vi "Go2XYZ (SubVI).vi"(0 ".NET Refnum in":refnum<k24>, 5 "Go to Coordinates":T2={"Go to X"=25.0, "Go to Y"=12.5, "Go to Z"=5.0}, 7 "Axis Speeds":T4={"X Speed"=25.0, "Y Speed"=12.5, "Z Speed"=5.0}, 11 "error in (no error)":errorcluster) -> (4 ".NET Refnum out":refnum<k24>, 6 "Final Position":T1, 14 "Initial Position":T3, 15 "error out":errorcluster)   [LabVIEW 2016]
uses:
  C:/Users/Aerotech/Documents/BNLStaveAssembly/Bin/Aerotech.A3200.dll
  Bin/Aerotech.A3200.dll
  Motion/EnableMultiple.vi
  Motion/MoveIncMultiple.vi
  Motion/WaitMultiple.vi
  Motion/DisableMultiple.vi
panel:
  out "Step Distance":dbl[](array[numeric])
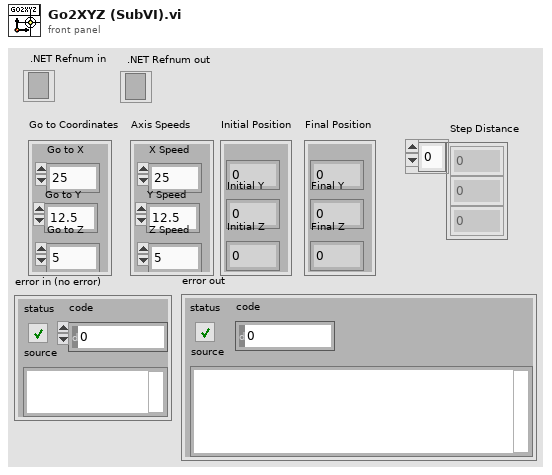
[diagram p1: front panel]
types:
  T1 = cluster{"Final X":dbl, "Final Y":dbl, "Final Z":dbl}
  T2 = cluster{"Go to X":dbl, "Go to Y":dbl, "Go to Z":dbl}
  T3 = cluster{"Initial X":dbl, "Initial Y":dbl, "Initial Z":dbl}
  T4 = cluster{"X Speed":dbl, "Y Speed":dbl, "Z Speed":dbl}
  T5 = cluster{"X Position Feedback":dbl, "Y Position Feedback":dbl, "Z Position Feedback":dbl}
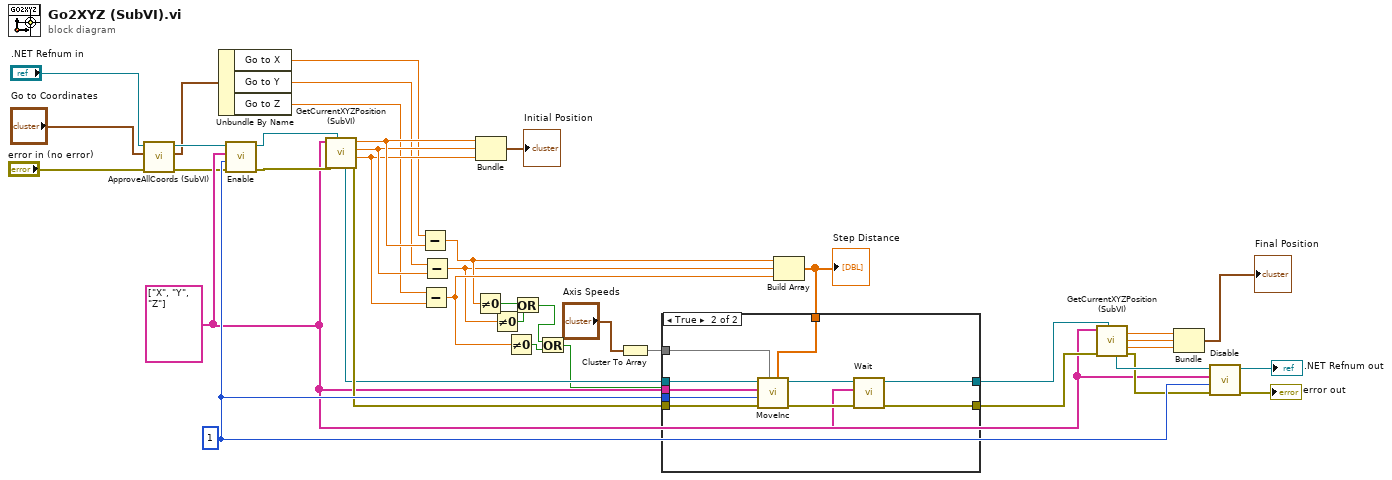
[diagram p0: block diagram]
diagram:
  w24 = string[] ["X", "Y", "Z"]
  w38 = 1 ("taskNumber")
  n1 = call "ApproveAllCoords (SubVI).vi"("error in (no error)"="error in (no error)", "Go to Coordinates"="Go to Coordinates", "Controller .NET Refnum in"=".NET Refnum in") -> ("error out"=w17:errorcluster, "Approved Coordinates"=w12:T2, "Controller .NET Refnum out"=w13:refnum<k24>)  [unwired: 6 in]
  n2 = Unbundle By Name(w12) -> ("Go to X"=w14:dbl, "Go to Y"=w15:dbl, "Go to Z"=w16:dbl)
  n3 = call-poly "Enable.vi"("error in (no error)"=w17, "taskId"=w38, "axis names"=w24, "controller in"=w13) -> ("error out"=w35:errorcluster, "controller out"=w34:refnum<k24>)  [unwired: 6 in]
  n4 = call "GetCurrentXYZPosition (SubVI).vi"(".NET Refnum in - Device"=w34, "error in (no error)"=w35, "Axes Names"=w24) -> ("error out"=w37:errorcluster, "Z Position Feedback"=w29:dbl, "Y Position Feedback"=w30:dbl, "X Position Feedback"=w31:dbl, ".NET Refnum out  - Device"=w36:refnum<k24>)  [unwired: 3 in]
  n5 = Subtract(x=w14, y=w31) -> (x-y=w7:dbl)
  n6 = Subtract(x=w16, y=w29) -> (x-y=w9:dbl)
  n7 = Subtract(x=w15, y=w30) -> (x-y=w6:dbl)
  n8 = Not Equal To 0?(x=w7) -> (x != 0?=w5:bool)
  n9 = Bundle("X Position Feedback"=w31, "Y Position Feedback"=w30, "Z Position Feedback"=w29) -> (→"Initial Position":T5)  [unwired: 1 in]
  n10 = Not Equal To 0?(x=w6) -> (x != 0?=w4:bool)
  n11 = Not Equal To 0?(x=w9) -> (x != 0?=w2:bool)
  n12 = Or(x=w5, y=w4) -> (x .or. y?=w3:bool)
  n13 = Or(x=w3, y=w2) -> (x .or. y?=w1:bool)
  n14 = Cluster To Array(cluster="Axis Speeds") -> (array=w32:dbl[])
  n15 = Build Array(w7, w6, w9) -> (w8:dbl[])
  "Step Distance" <- w8
  n16 = case shown="True" w1 {
    tunnel: w38 -> [_ w52]
    tunnel: w37 -> [w42 w49]
    tunnel: w36 -> [w41 w48]
    tunnel: w32 -> [_ w47]
    tunnel: [w41 w46] -> w28
    tunnel: [w42 w45] -> w26
    tunnel: w24 -> [_ w44]
    tunnel: w8 -> [_ w43]
    frame False {
    }
    frame True {
      n17 = call-poly "MoveInc.vi"("distances"=w43, "speeds"=w47, "error in (no error)"=w49, "taskId"=w52, "axis names"=w44, "controller in"=w48) -> ("error out"=w51:errorcluster, "controller out"=w50:refnum<k24>)  [unwired: 4 in]
      n18 = call-poly "Wait.vi"("error in (no error)"=w51, "axis names"=w44, "controller in"=w50) -> ("error out"=w45:errorcluster, "controller out"=w46:refnum<k24>)  [unwired: 6 in, 1 out]
    }
  }
  n19 = call "GetCurrentXYZPosition (SubVI).vi"(".NET Refnum in - Device"=w28, "error in (no error)"=w26, "Axes Names"=w24) -> ("error out"=w25:errorcluster, "Z Position Feedback"=w21:dbl, "Y Position Feedback"=w22:dbl, "X Position Feedback"=w23:dbl, ".NET Refnum out  - Device"=w27:refnum<k24>)  [unwired: 3 in]
  n20 = Bundle("X Position Feedback"=w23, "Y Position Feedback"=w22, "Z Position Feedback"=w21) -> (→"Final Position":T5)  [unwired: 1 in]
  n21 = call-poly "Disable.vi"("error in (no error)"=w25, "taskId"=w38, "axis names"=w24, "controller in"=w27) -> ("error out"=→"error out":errorcluster, "controller out"=→".NET Refnum out":refnum<k24>)  [unwired: 6 in]
